vi "Calc_T_tune_to_bydV.vi"(9 "dV":dbl=0.99999, 10 "T slave in":dbl=0.99999, 11 "T master in":dbl=0.99999) -> (2 "T slave tune to":dbl=97.72219547120214 format="%.3f", 3 "T master tune to":dbl=97.72219547120214 format="%.3g")   [LabVIEW 2010]
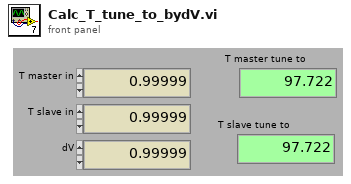
[diagram p1: front panel]
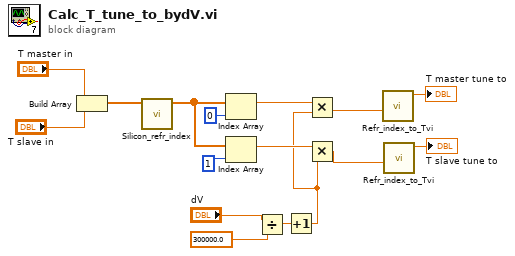
[diagram p0: block diagram]
diagram:
  n1 = Build Array("T master in", "T slave in") -> (w14:dbl[])
  n2 = call "Silicon_refr_index.vi"("Temperature"=w14) -> ("Silicon refr index at T"=w11:dbl[])  [unwired: 8 in, 2 out]
  n3 = Index Array(array=w11, index=0) -> (element=w7:dbl)
  n4 = Index Array(array=w11, index=1) -> (element=w6:dbl)
  n5 = Divide(x="dV", y=sgl 300000.0) -> (x/y=w8:dbl)
  n6 = Increment(x=w8) -> (x+1=w5:dbl)
  n7 = Multiply(x=w7, y=w5) -> (x*y=w4:dbl)
  n8 = Multiply(x=w6, y=w5) -> (x*y=w3:dbl)
  n9 = call "Refr_index_to_Tvi.vi"("refr inx"=w4) -> ("T tune to"=→"T master tune to":dbl)  [unwired: 9 in, 1 out]
  n10 = call "Refr_index_to_Tvi.vi"("refr inx"=w3) -> ("T tune to"=→"T slave tune to":dbl)  [unwired: 9 in, 1 out]
